vi "Show Image Window.vi"   [LabVIEW 2020, in "g_ar_toolkit.lvlib"]
uses:
  g_ar_toolkit.lvlib
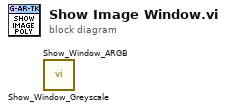
[diagram p0: block diagram]
diagram:
  n1 = call "Show_Window_Greyscale.vi"() -> ()  [unwired: 10 in, 2 out]
  n2 = call "Show_Window_ARGB.vi"() -> ()  [unwired: 10 in, 2 out]
